vi "Intake Modifications.vi"(1 "Intake Info In":T1, 2 "Cannon vbus":dbl) -> (0 "Intake Info In":T1)   [LabVIEW 2013]
panel:
  in  "t":dbl=1.05
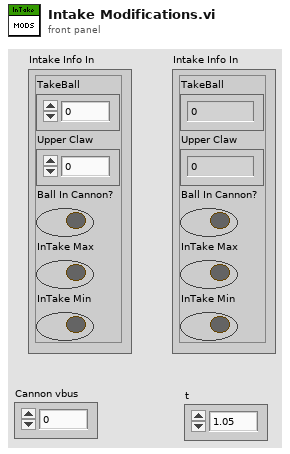
[diagram p1: front panel]
types:
  T1 = cluster{"TakeBall":dbl, "Upper Claw":dbl, "Ball In Cannon?":bool, "InTake Max":bool, "InTake Min":bool}
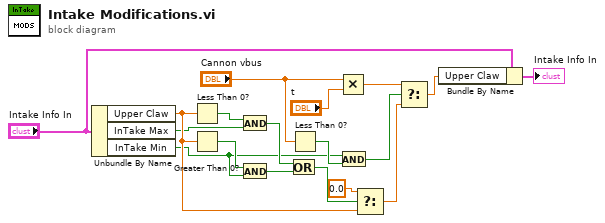
[diagram p0: block diagram]
diagram:
  n1 = Unbundle By Name("Intake Info In") -> ("Upper Claw"=w5:dbl, "InTake Max"=w4:bool, "InTake Min"=w1:bool)
  n2 = Less Than 0?(x=w5) -> (x < 0?=w6:bool)
  n3 = Greater Than 0?(x=w5) -> (x > 0?=w9:bool)
  n4 = And(x=w6, y=w4) -> (x .and. y?=w7:bool)
  n5 = And(x=w9, y=w1) -> (x .and. y?=w8:bool)
  n6 = Or(x=w7, y=w8) -> (x .or. y?=w10:bool)
  n7 = Less Than 0?(x="Cannon vbus") -> (x < 0?=w12:bool)
  n8 = Multiply(x="Cannon vbus", y="t") -> (x*y=w15:dbl)
  n9 = And(x=w1, y=w12) -> (x .and. y?=w13:bool)
  n10 = Select(t=0.0, s=w10, f=w5) -> (s? t:f=w16:dbl)
  n11 = Select(t=w15, s=w13, f=w16) -> (s? t:f=w3:dbl)
  n12 = Bundle By Name(cluster="Intake Info In", "Upper Claw"=w3) -> (→"Intake Info In":T1)
